vi "Test TIFF Write.vi"() -> ()   [LabVIEW 2020]
panel:
  out "Intensity Graph":u16[][](graph)
  in  "Path":path=path "D:/Data/Andor Test Videos/Pupil_23May16_120833.000.u16"
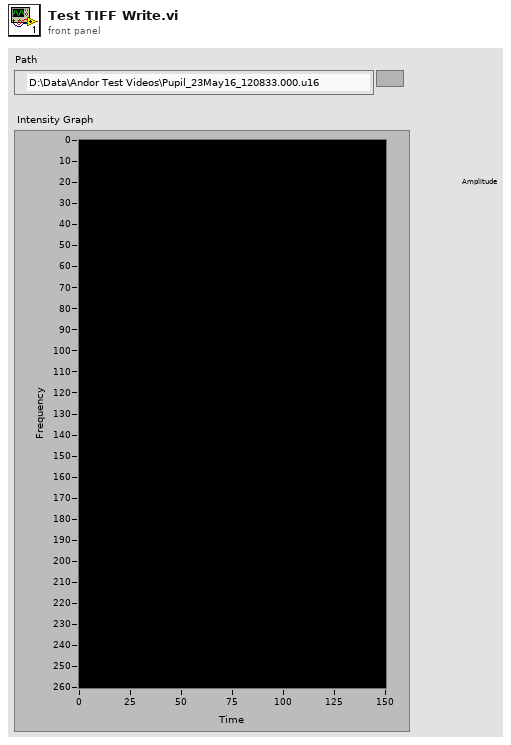
[diagram p1: front panel]
types:
  T1 = enum16{"open", "replace", "create", "open or create", "replace or create", "replace or create with confirmation"}
  T2 = typedef "TIFF-Write State.ctl" = cluster{"file":refnum<file>, "IFD":u8[], "offset":u32, "byte order":enum16{"big-endian, network order", "native, host order", "little-endian"}, "image size":u32, "IFD size":u32, "max frames":u32, "frames":u32}
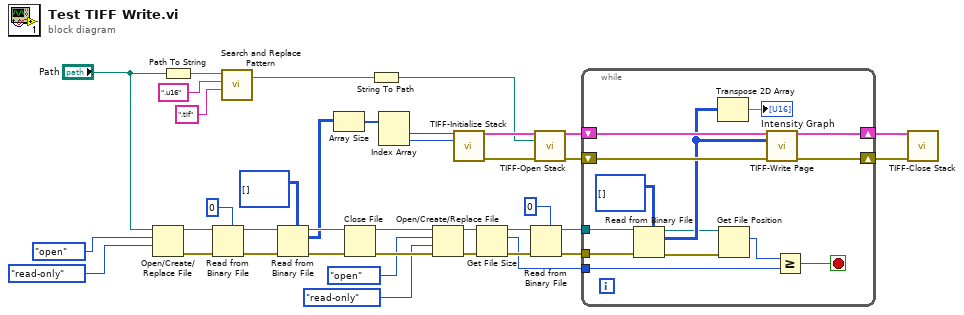
[diagram p0: block diagram]
diagram:
  n1 = Open/Create/Replace File(file path (use dialog)="Path", operation (0:open)=T1."open", access (0:read/write)=enum16{"read/write", "read-only", "write-only"}."read-only") -> (refnum out=w35:refnum<file>, error out=w36:errorcluster)  [unwired: 3 in, 1 out]
  n2 = Path To String(path="Path") -> (string=w27:string)
  n3 = Read from Binary File(5:0, 8:w36, 11:w35) -> (0:w33:errorcluster, 3:w32:refnum<file>)  [unwired: 3 in, 2 out]
  n4 = call <vilib>:"Search and Replace Pattern.vi"("string"=w27, "regular expression (\"\")"=".u16" ("regular expression (\"\")"), "replace string (\"\")"=".tif" ("replace string (\"\")")) -> ("result string"=w24:string)  [unwired: 2 in, 1 out]
  n5 = Read from Binary File(5:u16[][] [], 8:w33, 11:w32) -> (0:w30:errorcluster, 2:w15:u16[][], 3:w29:refnum<file>)  [unwired: 3 in, 1 out]
  n6 = Array Size(array=w15) -> (size(s)=w23:i32[])
  n7 = Close File(refnum=w29, error in=w30) -> (path=w14:path, error out=w13:errorcluster)
  n8 = String To Path(string=w24) -> (path=w18:path)
  n9 = Index Array(array=w23) -> (element #1=w22:i32, element #2=w21:i32)  [unwired: 2 in]
  n10 = Open/Create/Replace File(file path (use dialog)=w14, error in=w13, operation (0:open)=T1."open", access (0:read/write)=enum16{"read/write", "read-only", "write-only"}."read-only") -> (refnum out=w4:refnum<file>, error out=w3:errorcluster)  [unwired: 2 in, 1 out]
  n11 = call "TIFF-Initialize Stack.vi"("height"=w22, "width"=w21) -> ("state"=w19:T2, "error out"=w20:errorcluster)  [unwired: 12 in]
  n12 = Get File Size(file=w4, error in=w3) -> (refnum out=w2:refnum<file>, size (in bytes)=w1:i64, 0:w5:errorcluster)
  n13 = Read from Binary File(5:0, 8:w5, 11:w2) -> (0:w8:errorcluster, 3:w9:refnum<file>)  [unwired: 3 in, 2 out]
  n14 = call "TIFF-Open Stack.vi"("stack in"=w19, "file path (use dialog)"=w18, "error in"=w20) -> ("stack out"=w17:T2, "error out"=w16:errorcluster)  [unwired: 11 in]
  n15 = while {
    shift-right: [w50] -> w7
    shift-left: w17 -> [w52]
    shift-right: [w49] -> w6
    shift-left: w16 -> [w51]
    tunnel: w9 -> [w46]
    tunnel: w8 -> [w45]
    tunnel: w1 -> [w39]
    stop <- w40 stop-if-true
    n16 = Read from Binary File(5:u16[][] [], 8:w45, 11:w46) -> (0:w42:errorcluster, 2:w47:u16[][], 3:w43:refnum<file>)  [unwired: 3 in, 1 out]
    n17 = Transpose 2D Array(2D array=w47) -> (transposed array=→"Intensity Graph":u16[][])
    n18 = Get File Position(4:w42, 7:w43) -> (2:w41:i64)  [unwired: 2 out]
    n19 = call "TIFF-Write Page.vi"("state in"=w52, "Image Pixels (U16)"=w47, "error in"=w51) -> ("state out"=w50:T2, "error out"=w49:errorcluster)  [unwired: 11 in]
    n20 = Greater Or Equal?(x=w41, y=w39) -> (x >= y?=w40:bool)
  }
  n21 = call "TIFF-Close Stack.vi"("stack in"=w7, "error in"=w6) -> ()  [unwired: 12 in, 2 out]
